vi "Tag Write.vi"(2 "Tag array":refnum<class "NI Skyline Tag.lvclass">[](array[class]), 3 "Btuuon Value":string, 4 "i":i32, 5 "error in (no error)":errorcluster, 8 "Data":T2 {"RMS" format="%0.6f"; "RPM" format="%0.2f"; "Voltage" format="%0.2f"; "Current" format="%0.2f"; "Temperature" format="%0.2f"}) -> (19 "error out":errorcluster)   [LabVIEW 2017]
uses:
  typedefs/Data.ctl
  <vilib>/Skyline/Tag/Wrapper/Wrapper_class/NI Skyline Tag.lvclass
  <vilib>/Skyline/Tag/Wrapper/Wrapper_class/Tag Value Cluster Wrapper.ctl
  <vilib>/Skyline/Configuration/Configuration_class/NI Skyline Configuration.lvclass
  <vilib>/Skyline/Tag/Shared/typedefs/Tag Value Cluster.ctl
  <vilib>/Skyline/Tag/Shared/typedefs/DataType.ctl
  <vilib>/Skyline/Tag/Wrapper/Wrapper_class/Generate Tag Cluster (DBL) 2.vi
  <vilib>/Skyline/Tag/Wrapper/Wrapper_class/Generate Tag Cluster (String) 2.vi
  <vilib>/Skyline/Tag/Wrapper/Wrapper_class/Generate Tag Cluster (Boolean) 2.vi
  <vilib>/Skyline/Tag/Shared/NI Skyline Tag.lvlib
panel:
  in  "threshold cluster":T1={"RMS threshold"=2.0, "RPM threshold"=600000.0, "Voltage threshold"=0.0, "Current threshold"=0.0, "Temperature threshold"=20.0} {"Temperature threshold" format="%#_13g"; "Current threshold" format="%#_13g"; "Voltage threshold" format="%#_13g"; "RPM threshold" format="%#_13g"; "RMS threshold" format="%#_13g"}
  out "string write to table":string
  out "String":string
  # "RMS"
  # "RPM"
  # "Voltage"
  # "Current"
  # "Temper"
  # "Button"
  # "Table"
  # "Alarm"
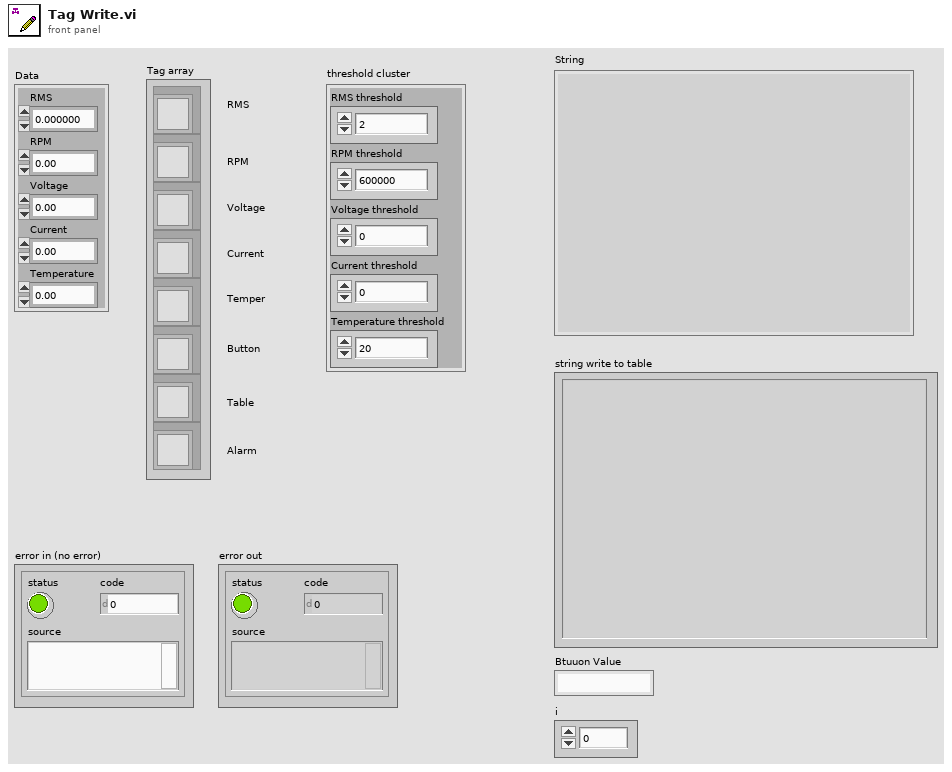
[diagram p1: front panel]
types:
  T1 = cluster{"RMS threshold":dbl, "RPM threshold":dbl, "Voltage threshold":dbl, "Current threshold":dbl, "Temperature threshold":dbl}
  T2 = typedef "Data.ctl" = cluster{"RMS":dbl, "RPM":dbl, "Voltage":dbl, "Current":dbl, "Temperature":dbl}
  T3 = typedef "NI Skyline Tag.lvclass/Tag Value Cluster Wrapper.ctl" = cluster{"Configuration":refnum<class "NI Skyline Configuration.lvclass">, "Tag Cluster":T4}
  T4 = typedef "NI Skyline Tag.lvlib/Tag Value Cluster.ctl" = cluster{"Path":string, "Data Type":T5, "Value":string, "Time Stamp":timestamp}
  T5 = typedef "NI Skyline Tag.lvlib/DataType.ctl" = enum32{"Double", "I32", "String", "Boolean", "U64", "Timestamp"}
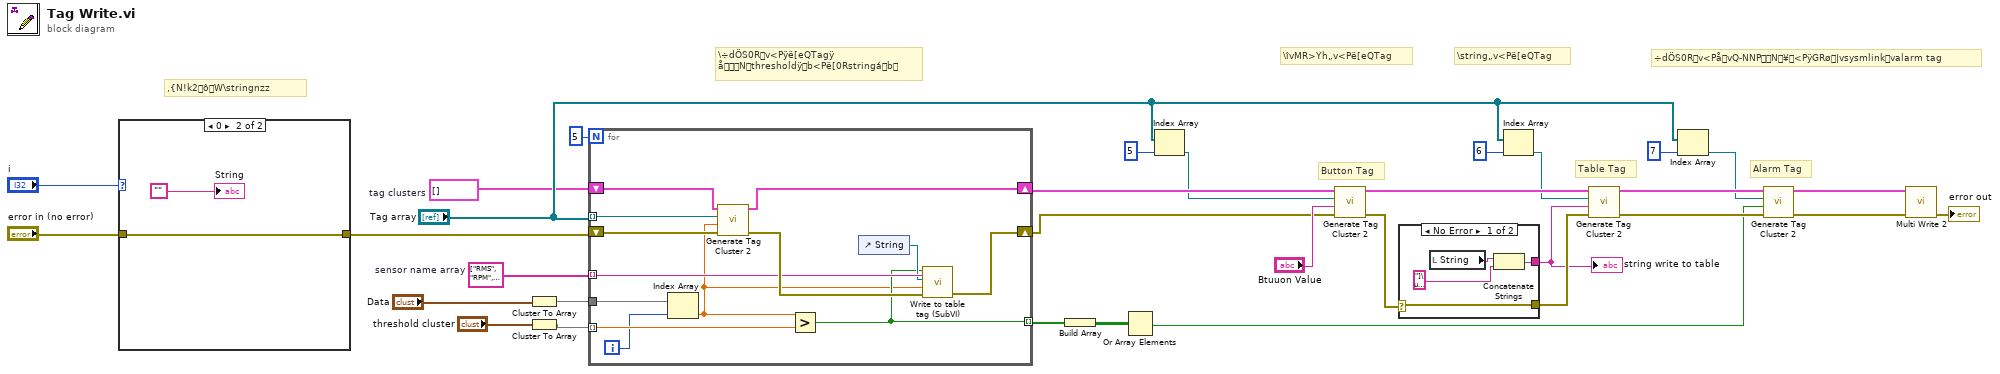
[diagram p0: block diagram]
diagram:
  w3 = T3[] []  # tag clusters
  w21 = string[] ["RMS", "RPM", "Voltage", "Current", "Temperature"]  # sensor name array
  # "\\string„v<Pë[eQTag"
  # "\\îvMR>Yh„v<Pë[eQTag"
  # "\\÷dÖS0Rv<Pÿë[eQTagÿ\nåNthresholdÿb<Pë[0Rstringáb"
  # ",{N!k2ôW\\stringnzz"
  # "÷dÖS0Rv<PåvQ-NNPN¥<PÿGRø|vsysmlinkvalarm tag"
  # "Alarm Tag"
  # "Table Tag"
  # "Button Tag"
  n1 = case shown="0" "i" {
    tunnel: [w33 w34] -> w15
    tunnel: "error in (no error)" -> [w33 w34]
    frame Default {
    }
    frame 0 {
      "String" <- ""
    }
  }
  n2 = Cluster To Array(cluster="Data") -> (array=w4:dbl[])
  n3 = Cluster To Array(cluster="threshold cluster") -> (array=w16:dbl[])
  n4 = for {
    N: 5 -> [_]
    tunnel: "Tag array" -> [w48] mode=indexing
    shift-right: [w47] -> w13
    shift-left: w3 -> [w45]
    shift-right: [w43] -> w14
    shift-left: w15 -> [w46]
    tunnel: w21 -> [w42] mode=indexing
    tunnel: w16 -> [w40] mode=indexing
    tunnel: [w39] -> w19 mode=indexing
    tunnel: w4 -> [w37]
    i -> [w38]
    n5 = Index Array(array=w37, index=w38) -> (element=w36:dbl)
    n6 = call-poly <vilib>:"Generate Tag Cluster 2.vi"("error in (no error)"=w46, "value"=w36, "tag in"=w48, "tag clusters in"=w45) -> ("error out"=w44:errorcluster, "tag clusters out"=w47:T3[])  [unwired: 5 in, 1 out]
    n7 = Greater?(x=w36, y=w40) -> (0:w39:bool)
    n8 = control-ref of="String"() -> (w41:refnum<vi>)
    n9 = call "Write to table tag (SubVI).vi"("alarm?"=w39, "Sensor Name"=w42, "table value"=w41, "Sensor Value"=w36, "error in (no error)"=w44) -> ("error IO"=w43:errorcluster)  [unwired: 3 in]
  }
  n10 = Build Array(w19) -> (w18:bool[][])
  n11 = Or Array Elements(Boolean array=w18) -> (logical OR=w1:bool)
  n12 = Index Array(array="Tag array", index=5) -> (element=w9:refnum<class "NI Skyline Tag.lvclass">)
  n13 = call-poly <vilib>:"Generate Tag Cluster 2.vi"("error in (no error)"=w14, "value"="Btuuon Value", "tag in"=w9, "tag clusters in"=w13) -> ("error out"=w29:errorcluster, "tag clusters out"=w30:T3[])  [unwired: 5 in, 1 out]
  n14 = case shown="No Error" w29 {
    selector: w29 -> [w49 w53]
    tunnel: [w51 _] -> w27
    tunnel: [w49 w53] -> w28
    frame No Error {
      n15 = local read "String"() -> (w52:string)
      n16 = Concatenate Strings(w52, "]\u0000" ("string")) -> (w51:string)
    }
    frame Error {
    }
  }
  "string write to table" <- w27
  n17 = Index Array(array="Tag array", index=6) -> (element=w8:refnum<class "NI Skyline Tag.lvclass">)
  n18 = call-poly <vilib>:"Generate Tag Cluster 2.vi"("error in (no error)"=w28, "value"=w27, "tag in"=w8, "tag clusters in"=w30) -> ("error out"=w25:errorcluster, "tag clusters out"=w26:T3[])  [unwired: 5 in, 1 out]
  n19 = Index Array(array="Tag array", index=7) -> (element=w6:refnum<class "NI Skyline Tag.lvclass">)
  n20 = call-poly <vilib>:"Generate Tag Cluster 2.vi"("error in (no error)"=w25, "value"=w1, "tag in"=w6, "tag clusters in"=w26) -> ("error out"=w23:errorcluster, "tag clusters out"=w24:T3[])  [unwired: 5 in, 1 out]
  n21 = call <vilib>:"Multi Write 2.vi"("error in (no error)"=w23, "tag clusters"=w24) -> ("error out"=→"error out":errorcluster)  [unwired: 9 in]
